vi "Autonomous Independent.vi"   [LabVIEW 2014]
doc: "This VI is called when autonomous begins, and will automatically be terminated when autonomous ends. You can carry out timed or sensor driven robot movement independently without needing to return to the caller."
panel:
  # "Be sure to right-click and choose Data Operations>>Make Current Value default if you want to save the array values with the VI"
types:
  T1 = typedef "Autonomous Play Definition.ctl" = cluster{"Play Name":string, "Command List":cluster{"Param 1":dbl, "Param 2":dbl, "Autonomous Command Name":T2, "Concurrent":bool}[], "Play Description":string}
  T2 = typedef "Autonomous Command Names.ctl" = enum16{"No Op", "Drive Distance Robot", "Drive Time Robot", "Translate Distance Robot", "Translate Time Robot", "Drive Distance Field", "Drive Time Field", "Translate Distance Field", "Translate Time Field", "Rotate Robot", "Set Initial Gyro Value", "Lifter to Setpoint", "Wait", "Do Not use", "Drive Distance Field (Gyro Hold)", "Translate Distance Field (Gyro Hold)", "Can", "Grabber", "Drive Distance Field (Sensor Stop, Gyro Hold)", "Move Direction Field (Gyro Hold)", "Rotate Robot 90 about Tote", "Reset Gyro", "Find Tote", "Get Tote Into Robot", "Lower Can Grabber"}
  T3 = typedef "Robot Commands.ctl" = cluster{"Robot Forward-Reverse":dbl, "Robot Left-Right":dbl, "Robot Twist":dbl, "Can Load Mode Enabled":bool, "Lifter in Manual Override?":bool, "Stack Drop Command":bool, "Arm Raised?":bool, "DISABLE LIFTER":bool, "Position 1 Setpoint":bool, "Position 2 Setpoint":bool, "Position 3 Setpoint":bool, "Position 4 Setpoint":bool, "Position 5 Setpoint":bool, "Bump Lifter Down":bool, "Bump Lifter Up":bool, "Manual Load Command":bool, "Robot Centric?":bool, "Scissor Deploy/Retract":bool, "Grabber":bool, "Can":bool, "Twist arm up":bool, "Gyro Reset":bool, "Twist arm down":bool, "Short Sequence Load":bool, "Robot Twist X":dbl, "Robot Twist Y":dbl}
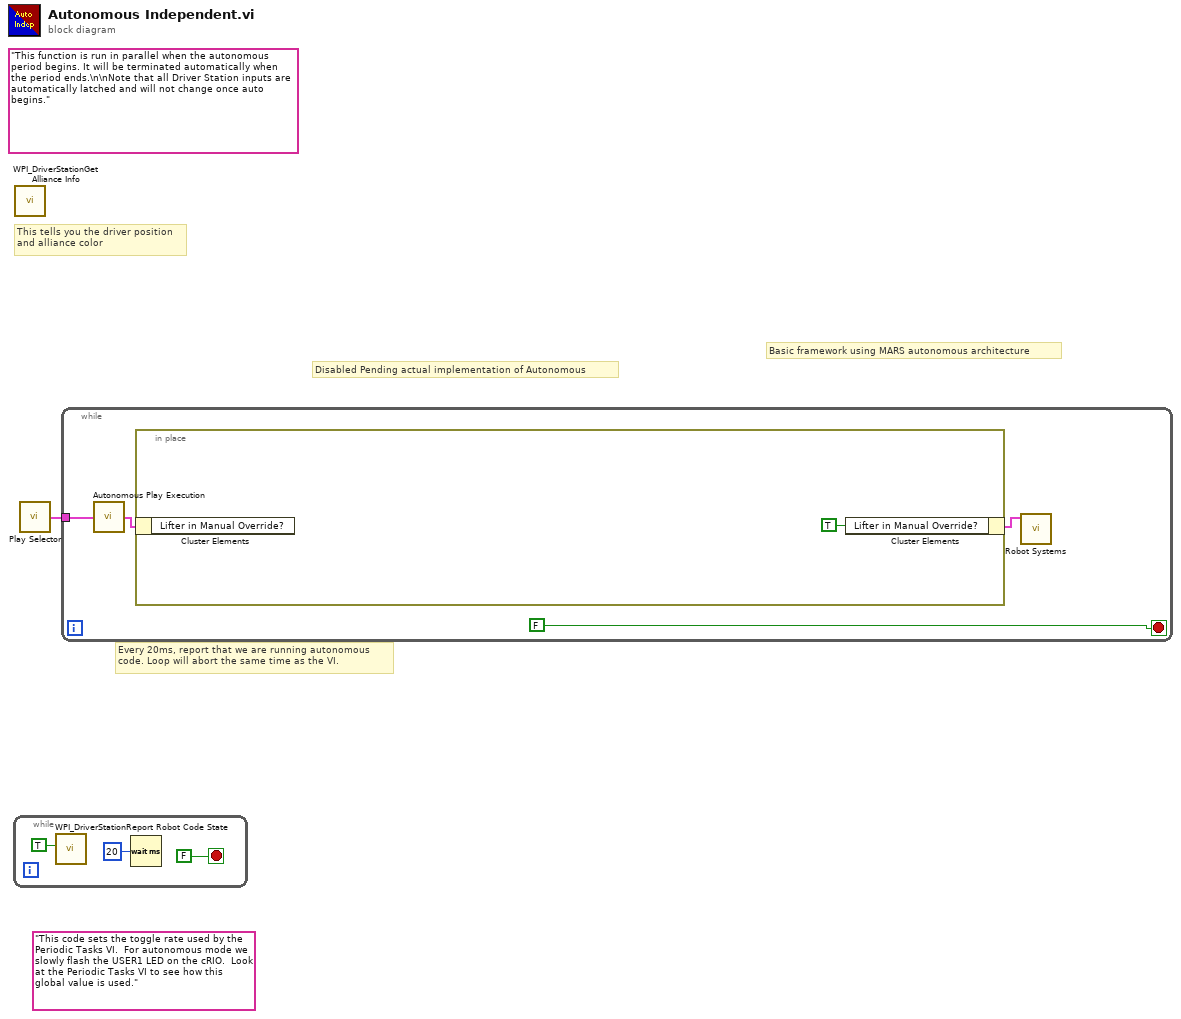
[diagram p0: block diagram]
diagram:
  (unwired) "This code sets the toggle rate used by the Periodic Tasks VI.  For autonomous mode we slowly flash the USER1 LED on the cRIO.  Look at the Periodic Tasks VI to see how this global value is used."
  (unwired) "This function is run in parallel when the autonomous period begins. It will be terminated automatically when the period ends.\n\nNote that all Driver Station inputs are automatically latched and will not change once auto begins."
  # "Disabled Pending actual implementation of Autonomous"
  # "Basic framework using MARS autonomous architecture"
  # "Every 20ms, report that we are running autonomous\ncode. Loop will abort the same time as the VI."
  # "This tells you the driver position\nand alliance color"
  n1 = while {
    stop <- FALSE stop-if-true
    n2 = call <vilib>:"WPI_DriverStationReport Robot Code State.vi"("Autonomous"=TRUE) -> ()  [unwired: 10 in, 1 out]
    n3 = Wait (ms)(milliseconds to wait=u32 20) -> ()  [unwired: 1 out]
  }
  n4 = call <vilib>:"WPI_DriverStationGet Alliance Info.vi"() -> ()  [unwired: 12 out]
  n5 = call "Play Selector.vi"() -> ("Output Play"=w1:T1)  [unwired: 1 in]
  n6 = while {
    tunnel: w1 -> [w7]
    stop <- FALSE stop-if-true
    n7 = call "Autonomous Play Execution.vi"("Input Play"=w7) -> ("Robot System Functions"=w6:T3)
    n8 = in-place {
      n9 = in-place-cluster #1(w6) -> ()  [unwired: 1 out]
      n10 = in-place-cluster #1("Lifter in Manual Override?"=TRUE) -> (w5:T3)
    }
    n11 = call "Robot Systems.vi"("Robot Controls"=w5) -> ()  [unwired: 11 in]
  }
